vi "S2C_ExeScriptUpdateEvent.vi"(8 "Error In":errorcluster, 11 "Result":string) -> (0 "Error Out":errorcluster)   [LabVIEW 2015]
doc: "Determines the result for the currently executing line item, and updates the measurement and result in the data array."
uses:
  Controls/S2C_ResultStatus.ctl
  Globals/S2C_Globals.vi
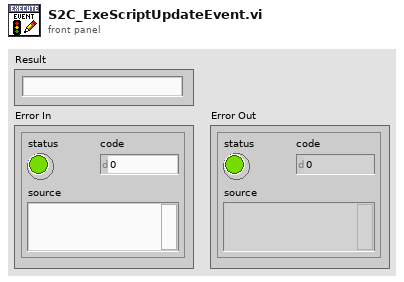
[diagram p1: front panel]
types:
  T1 = typedef "S2C_ResultStatus.ctl" = enum16{"Passed", "Failed", "Logged", "Aborted", "Error", "Testing...", "Paused", "No Record"}
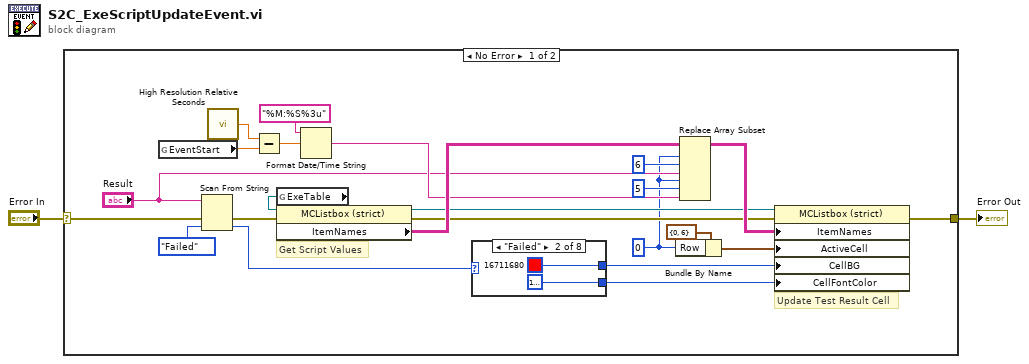
[diagram p0: block diagram]
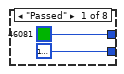
[diagram p2: hidden frame]
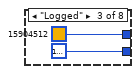
[diagram p3: hidden frame]
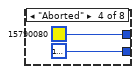
[diagram p4: hidden frame]
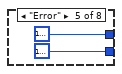
[diagram p5: hidden frame]
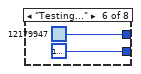
[diagram p6: hidden frame]
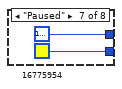
[diagram p7: hidden frame]
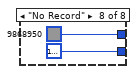
[diagram p8: hidden frame]
diagram:
  n1 = case shown="No Error" "Error In" {
    selector: "Error In" -> [w5 w42]
    tunnel: [w25 w42] -> w1
    frame No Error {
      w3 = 0 ("disabled index (col)")
      # "Update Test Result Cell"
      # "Get Script Values"
      n2 = global read "S2C_Globals.vi" "EventStart"() -> (w10:dbl)
      n3 = Scan From String(input string="Result", error in=w5, default 1=S2C_ResultStatus."Failed" ("y")) -> (error out=w17:errorcluster, output 1=w16:T1)  [unwired: 2 in, 2 out]
      n4 = call <vilib>:"High Resolution Relative Seconds.vi"() -> ("relative seconds"=w11:dbl)
      n5 = Subtract(x=w11, y=w10) -> (x-y=w9:dbl)
      n6 = global read "S2C_Globals.vi" "ExeTable"() -> (w18:refnum<vi>)
      n7 = property class="MCListbox (strict)"(reference=w18, error in=w17) -> (reference out=w13:refnum<vi>, error out=w15:errorcluster, "ItemNames"=w19:string[][])
      n8 = Format Date/Time String(time format string (%c)="%M:%S%3u", seconds (now)=w9) -> (date/time string=w6:string)  [unwired: 1 in]
      n9 = case shown="\"Failed\"" w16 {
        tunnel: [u32 46081 u32 16711680 u32 15904512 u32 15790080 u32 16777222 u32 12179947 u32 16777222 u32 9868950] -> w20
        tunnel: [u32 16777226 u32 16777226 u32 16777226 u32 16777222 u32 16777226 u32 16777222 u32 16775954 u32 16777226] -> w14
        frame "Passed" {
        }
        frame "Failed" {
        }
        frame "Logged" {
        }
        frame "Aborted" {
        }
        frame "Error" {
        }
        frame "Testing..." {
        }
        frame "Paused" {
        }
        frame "No Record" {
        }
      }
      n10 = Bundle By Name(cluster=cluster{"Row":i32, "Column":i32} {"Row"=0, "Column"=6} ("Active Cell:Active Cell"), "Row"=w3) -> (w21:cluster{"Row":i32, "Column":i32})
      n11 = Replace Array Subset(array=w19, new element #1="Result", index (row) #1=w3, index (col) #1=6 ("disabled index (col)"), new element #2=w6, index (row) #2=w3, index (col) #2=5 ("disabled index (col)")) -> (w23:string[][])
      n12 = property on="Property Node" class="MCListbox (strict)"(reference=w13, error in=w15, "ItemNames"=w23, "ActiveCell"=w21, "CellBG"=w20, "CellFontColor"=w14) -> (error out=w25:errorcluster)  [unwired: 1 out]
    }
    frame Error {
    }
  }
  "Error Out" <- w1
